vi "Wait Message Loop.vi"(8 "error in (no error)":errorcluster, 11 "Message Queues":T1) -> (0 "error out":errorcluster)   [LabVIEW 2023, in "Weather Wait Loop.lvlib"]
doc: "Message loop for waiting a period of time before signaling to start a request for weather updates."
uses:
  Weather Wait Loop.lvlib
  support/Message Queue/All Message Queues.ctl
  support/Message Queue/Message Cluster.ctl
  support/Message Queue/Weather Message Queue.lvlib
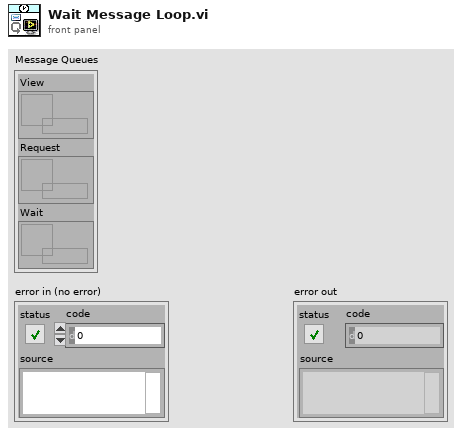
[diagram p1: front panel]
types:
  T1 = typedef "Weather Message Queue.lvlib/All Message Queues.ctl" = cluster{"View":refnum<queue>, "Request":refnum<queue>, "Wait":refnum<queue>}
  T2 = typedef "Weather Wait Loop.lvlib/User Events.ctl" = cluster{"Stop":refnum<user-event>, "Set Timeout":refnum<user-event>}
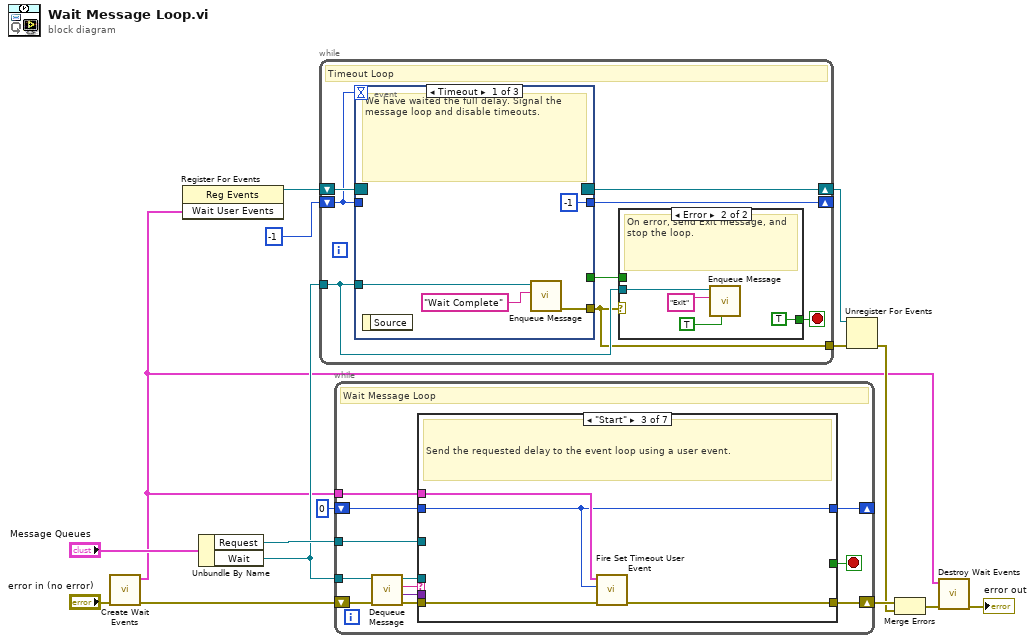
[diagram p0: block diagram]
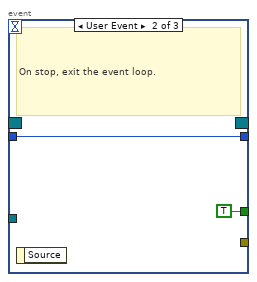
[diagram p3: hidden frame]
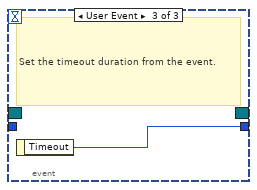
[diagram p4: hidden frame]
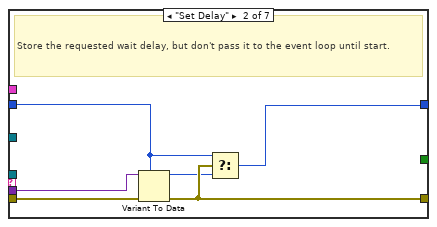
[diagram p6: hidden frame]
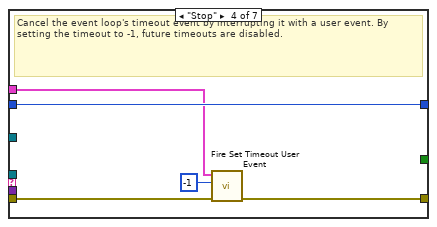
[diagram p7: hidden frame]
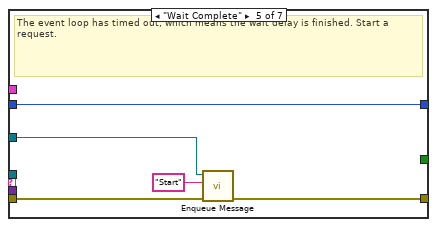
[diagram p8: hidden frame]
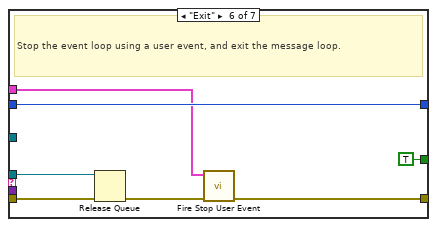
[diagram p9: hidden frame]
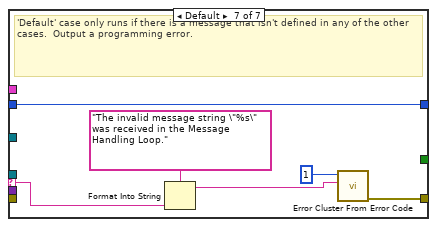
[diagram p10: hidden frame]
diagram:
  n1 = call "Create Wait Events.vi"("error in (no error)"="error in (no error)") -> ("error out"=w13:errorcluster, "Wait User Events"=w2:T2)  [unwired: 9 in]
  n2 = register-events(w2) -> (reference out=w1:refnum<event-registration>)  [unwired: 2 in, 1 out]
  n3 = Unbundle By Name("Message Queues") -> ("Request"=w8:refnum<queue>, "Wait"=w5:refnum<queue>)
  n4 = while {
    shift-right: [w21] -> _
    shift-left: -1 ("Timeout") -> [w20]
    tunnel: w5 -> [w17]
    shift-right: [w23] -> w12
    shift-left: w1 -> [w22]
    tunnel: [w16] -> w3
    stop <- w19 stop-if-true
    # "Timeout Loop"
    n5 = event shown="[0] Timeout" {
      selector: w22 -> [_ _ _]
      dyn-events: [_ _ _] -> w23
      timeout: w20 -> [_ _ _]
      tunnel: [-1 ("Timeout") w34 w35] -> w21
      tunnel: w20 -> [_ w34 _]
      tunnel: [_ TRUE _] -> w18
      tunnel: w17 -> [w32 _ _]
      tunnel: [w30 _ _] -> w16
      event Timeout {
        # "We have waited the full delay. Signal the message loop and disable timeouts."
        n6 = event-data() -> ()  [unwired: 1 in, 1 out]
        n7 = call "Enqueue Message.vi"("Message"="Wait Complete", "Message Queue"=w32) -> ("error out"=w30:errorcluster)  [unwired: 8 in, 1 out]
      }
      event User Event {
        # "On stop, exit the event loop."
        n8 = event-data() -> ()  [unwired: 1 in, 1 out]
      }
      event User Event {
        # "Set the timeout duration from the event."
        n9 = event-data() -> ("Timeout"=w35:i32)  [unwired: 1 in]
      }
    }
    n10 = case shown="Error" w16 {
      tunnel: [w24 TRUE] -> w19
      tunnel: w18 -> [w24 _]
      tunnel: w17 -> [_ w25]
      frame No Error {
      }
      frame Error {
        # "On error, send Exit message, and stop the loop."
        n11 = call "Enqueue Message.vi"("Priority Message? (F)"=TRUE ("Discard?"), "Message"="Exit", "Message Queue"=w25) -> ()  [unwired: 7 in, 2 out]
      }
    }
  }
  n12 = while {
    shift-right: [w39] -> w10
    shift-left: w13 -> [w46]
    tunnel: w8 -> [w37]
    tunnel: w5 -> [w47]
    shift-right: [w40] -> _
    shift-left: 0 ("Delay") -> [w41]
    tunnel: w2 -> [w36]
    stop <- w38 stop-if-true
    # "Wait Message Loop"
    n13 = call "Dequeue Message.vi"("error in (no error)"=w46, "Message Queue"=w47) -> ("error out"=w43:errorcluster, "Message Data"=w42:variant, "Message"=w45:string, "dup Message Queue"=w44:refnum<queue>)  [unwired: 6 in]
    n14 = case shown="\"Start\"" w45 {
      selector: w45 -> [_ _ _ _ _ _ w77]
      tunnel: w44 -> [_ _ _ _ _ w70 _]
      tunnel: w43 -> [w49 w55 w59 w63 w68 w75 _]
      tunnel: w42 -> [_ w54 _ _ _ _ _]
      tunnel: w41 -> [w48 w52 w56 w64 w69 w76 w82]
      tunnel: [w48 w50 w56 w64 w69 w76 w82] -> w40
      tunnel: [w49 w53 w58 w62 w67 w73 w78] -> w39
      tunnel: [_ _ _ _ _ TRUE _] -> w38
      tunnel: w37 -> [_ _ _ _ w66 _ _]
      tunnel: w36 -> [_ _ w57 w61 _ w72 _]
      frame "Initialize" {
        # "No additional initialization to do."
      }
      frame "Set Delay" {
        # "Store the requested wait delay, but don't pass it to the event loop until start."
        n15 = Variant To Data(error in=w55, type=w52, Variant=w54) -> (data=w51:i32, error out=w53:errorcluster)
        n16 = Select(t=w52, s=w53, f=w51) -> (s? t:f=w50:i32)
      }
      frame "Start" {
        # "Send the requested delay to the event loop using a user event."
        n17 = call "Fire Set Timeout User Event.vi"("error in (no error)"=w59, "Timeout"=w56, "Wait User Events"=w57) -> ("error out"=w58:errorcluster)  [unwired: 8 in]
      }
      frame "Stop" {
        # "Cancel the event loop's timeout event by interrupting it with a user event. By setting the timeout to -1, future timeouts are disabled."
        n18 = call "Fire Set Timeout User Event.vi"("error in (no error)"=w63, "Timeout"=-1, "Wait User Events"=w61) -> ("error out"=w62:errorcluster)  [unwired: 8 in]
      }
      frame "Wait Complete" {
        # "The event loop has timed out, which means the wait delay is finished. Start a request."
        n19 = call "Enqueue Message.vi"("error in (no error)"=w68, "Message"="Start", "Message Queue"=w66) -> ("error out"=w67:errorcluster)  [unwired: 7 in, 1 out]
      }
      frame "Exit" {
        # "Stop the event loop using a user event, and exit the message loop."
        n20 = Release Queue(queue=w70, error in (no error)=w75) -> (error out=w71:errorcluster)  [unwired: 1 in, 2 out]
        n21 = call "Fire Stop User Event.vi"("error in (no error)"=w71, "Wait User Events"=w72) -> ("error out"=w73:errorcluster)  [unwired: 9 in]
      }
      frame Default {
        # "'Default' case only runs if there is a message that isn't defined in any of the other cases.  Output a programming error."
        n22 = Format Into String(format string="The invalid message string \"%s\" was received in the Message Handling Loop." ("Unknown Message Error Text"), w77) -> (resulting string=w79:string)  [unwired: 2 in, 1 out]
        n23 = call <vilib>:"Error Cluster From Error Code.vi"("error message (\"\")"=w79, "error code (0)"=1) -> ("error out"=w78:errorcluster)  [unwired: 7 in]
      }
    }
  }
  n24 = Unregister For Events(event registration refnum=w12, error in=w3) -> (error out=w9:errorcluster)
  n25 = Merge Errors(w10, w9) -> (w11:errorcluster)
  n26 = call "Destroy Wait Events.vi"("error in (no error)"=w11, "Wait User Events"=w2) -> ("error out"=→"error out":errorcluster)  [unwired: 9 in]
